vi "Main_09b refactored.vi"() -> ()   [LabVIEW 2020]
uses:
  Cluster_Point.ctl
panel:
  in  "Puzzle Description":string="--- Part Two ---\nA rope snaps! Suddenly, the river is getting a lot closer than you remember. The bridge is still there, but some of the ropes that broke are now whipping toward you as you fall through the air!\n\nThe ropes are moving too quickly to grab; you only have a few seconds to choose how to arch your body to avoid being hit. Fortunately, your simulation can be extended to support longer ropes.\n\nRather than two knots, you now must simulate a rope consisting of ten knots. One knot is still the head of the rope and moves according to the series of motions. Each knot further down the rope follows the knot in front of it using the same rules as before.\n\nUsing the same series of motions as the above example, but with the knots marked H, 1, 2, ..., 9, the motions now occur as follows:\n\n== Initial State ==\n\n......\n......\n......\n......\nH.....  (H covers 1, 2, 3, 4, 5, 6, 7, 8, 9, s)\n\n== R 4 ==\n\n......\n......\n......\n......\n1H....  (1 covers 2, 3, 4, 5, 6, 7, 8, 9, s)\n\n......\n......\n......\n......\n21H...  (2 covers 3, 4, 5, 6, 7, 8, 9, s)\n\n......\n......\n......\n......\n321H..  (3 covers 4, 5, 6, 7, 8, 9, s)\n\n......\n......\n......\n......\n4321H.  (4 covers 5, 6, 7, 8, 9, s)\n\n== U 4 ==\n\n......\n......\n......\n....H.\n4321..  (4 covers 5, 6, 7, 8, 9, s)\n\n......\n......\n....H.\n.4321.\n5.....  (5 covers 6, 7, 8, 9, s)\n\n......\n....H.\n....1.\n.432..\n5.....  (5 covers 6, 7, 8, 9, s)\n\n....H.\n....1.\n..432.\n.5....\n6.....  (6 covers 7, 8, 9, s)\n\n== L 3 ==\n\n...H..\n....1.\n..432.\n.5....\n6.....  (6 covers 7, 8, 9, s)\n\n..H1..\n...2..\n..43..\n.5....\n6.....  (6 covers 7, 8, 9, s)\n\n.H1...\n...2..\n..43..\n.5....\n6.....  (6 covers 7, 8, 9, s)\n\n== D 1 ==\n\n..1...\n.H.2..\n..43..\n.5....\n6.....  (6 covers 7, 8, 9, s)\n\n== R 4 ==\n\n..1...\n..H2..\n..43..\n.5....\n6.....  (6 covers 7, 8, 9, s)\n\n..1...\n...H..  (H covers 2)\n..43..\n.5....\n6.....  (6 covers 7, 8, 9, s)\n\n......\n...1H.  (1 covers 2)\n..43..\n.5....\n6.....  (6 covers 7, 8, 9, s)\n\n......\n...21H\n..43..\n.5....\n6.....  (6 covers 7, 8, 9, s)\n\n== D 1 ==\n\n......\n...21.\n..43.H\n.5....\n6.....  (6 covers 7, 8, 9, s)\n\n== L 5 ==\n\n......\n...21.\n..43H.\n.5....\n6.....  (6 covers 7, 8, 9, s)\n\n......\n...21.\n..4H..  (H covers 3)\n.5....\n6.....  (6 covers 7, 8, 9, s)\n\n......\n...2..\n..H1..  (H covers 4; 1 covers 3)\n.5....\n6.....  (6 covers 7, 8, 9, s)\n\n......\n...2..\n.H13..  (1 covers 4)\n.5....\n6.....  (6 covers 7, 8, 9, s)\n\n......\n......\nH123..  (2 covers 4)\n.5....\n6.....  (6 covers 7, 8, 9, s)\n\n== R 2 ==\n\n......\n......\n.H23..  (H covers 1; 2 covers 4)\n.5....\n6.....  (6 covers 7, 8, 9, s)\n\n......\n......\n.1H3..  (H covers 2, 4)\n.5....\n6.....  (6 covers 7, 8, 9, s)\nNow, you need to keep track of the positions the new tail, 9, visits. In this example, the tail never moves, and so it only visits 1 position. However, be careful: more types of motion are possible than before, so you might want to visually compare your simulated rope to the one above.\n\nHere's a larger example:\n\nR 5\nU 8\nL 8\nD 3\nR 17\nD 10\nL 25\nU 20\nThese motions occur as follows (individual steps are not shown):\n\n== Initial State ==\n\n..........................\n..........................\n..........................\n..........................\n..........................\n..........................\n..........................\n..........................\n..........................\n..........................\n..........................\n..........................\n..........................\n..........................\n..........................\n...........H..............  (H covers 1, 2, 3, 4, 5, 6, 7, 8, 9, s)\n..........................\n..........................\n..........................\n..........................\n..........................\n\n== R 5 ==\n\n..........................\n..........................\n..........................\n..........................\n..........................\n..........................\n..........................\n..........................\n..........................\n..........................\n..........................\n..........................\n..........................\n..........................\n..........................\n...........54321H.........  (5 covers 6, 7, 8, 9, s)\n..........................\n..........................\n..........................\n..........................\n..........................\n\n== U 8 ==\n\n..........................\n..........................\n..........................\n..........................\n..........................\n..........................\n..........................\n................H.........\n................1.........\n................2.........\n................3.........\n...............54.........\n..............6...........\n.............7............\n............8.............\n...........9..............  (9 covers s)\n..........................\n..........................\n..........................\n..........................\n..........................\n\n== L 8 ==\n\n..........................\n..........................\n..........................\n..........................\n..........................\n..........................\n..........................\n........H1234.............\n............5.............\n............6.............\n............7.............\n............8.............\n............9.............\n..........................\n..........................\n...........s..............\n..........................\n..........................\n..........................\n..........................\n..........................\n\n== D 3 ==\n\n..........................\n..........................\n..........................\n..........................\n..........................\n..........................\n..........................\n..........................\n.........2345.............\n........1...6.............\n........H...7.............\n............8.............\n............9.............\n..........................\n..........................\n...........s..............\n..........................\n..........................\n..........................\n..........................\n..........................\n\n== R 17 ==\n\n..........................\n..........................\n..........................\n..........................\n..........................\n..........................\n..........................\n..........................\n..........................\n..........................\n................987654321H\n..........................\n..........................\n..........................\n..........................\n...........s..............\n..........................\n..........................\n..........................\n..........................\n..........................\n\n== D 10 ==\n\n..........................\n..........................\n..........................\n..........................\n..........................\n..........................\n..........................\n..........................\n..........................\n..........................\n..........................\n..........................\n..........................\n..........................\n..........................\n...........s.........98765\n.........................4\n.........................3\n.........................2\n.........................1\n.........................H\n\n== L 25 ==\n\n..........................\n..........................\n..........................\n..........................\n..........................\n..........................\n..........................\n..........................\n..........................\n..........................\n..........................\n..........................\n..........................\n..........................\n..........................\n...........s..............\n..........................\n..........................\n..........................\n..........................\nH123456789................\n\n== U 20 ==\n\nH.........................\n1.........................\n2.........................\n3.........................\n4.........................\n5.........................\n6.........................\n7.........................\n8.........................\n9.........................\n..........................\n..........................\n..........................\n..........................\n..........................\n...........s..............\n..........................\n..........................\n..........................\n..........................\n..........................\n\nNow, the tail (9) visits 36 positions (including s) at least once:\n\n..........................\n..........................\n..........................\n..........................\n..........................\n..........................\n..........................\n..........................\n..........................\n#.........................\n#.............###.........\n#............#...#........\n.#..........#.....#.......\n..#..........#.....#......\n...#........#.......#.....\n....#......s.........#....\n.....#..............#.....\n......#............#......\n.......#..........#.......\n........#........#........\n.........########.........\nSimulate your complete series of motions on a larger rope with ten knots. How many positions does the tail of the rope visit at least once?"
  out "Location array":T1[](array[typedef])
  in  "Example 1":string="R 4\nU 4\nL 3\nD 1\nR 4\nD 1\nL 5\nR 2"
  out "Tail Positon count":i32
  in  "Puzzle":string="R 1\nD 1\nL 1\nD 1\nR 2\nL 1\nU 2\nD 1\nU 2\nL 1\nU 1\nL 2\nD 1\nU 2\nL 1\nR 1\nD 1\nL 2\nD 2\nL 2\nR 1\nL 2\nU 2\nR 2\nL 2\nU 2\nL 1\nD 1\nL 2\nU 1\nR 1\nD 2\nL 2\nU 1\nR 1\nD 1\nU 2\nL 1\nD 2\nU 1\nD 1\nR 2\nD 1\nL 2\nD 1\nL 1\nR 1\nD 2\nL 1\nR 2\nD 2\nU 2\nR 2\nD 2\nR 2\nL 2\nD 2\nL 2\nD 1\nU 2\nR 1\nD 2\nL 2\nR 2\nL 1\nD 1\nU 2\nD 1\nR 2\nU 2\nR 2\nD 1\nL 1\nU 2\nD 1\nU 1\nD 2\nU 1\nR 1\nU 2\nD 1\nL 2\nU 1\nL 2\nD 2\nR 1\nU 2\nL 1\nD 2\nR 1\nU 1\nD 1\nL 2\nU 1\nR 1\nD 2\nU 2\nL 1\nU 2\nD 2\nR 1\nU 2\nR 1\nU 2\nR 1\nD 2\nU 1\nD 2\nL 2\nD 2\nL 2\nD 2\nR 1\nU 1\nD 3\nU 1\nR 2\nU 3\nD 1\nU 2\nD 2\nU 2\nD 1\nU 2\nR 2\nL 2\nU 1\nL 3\nD 1\nR 3\nD 3\nR 2\nL 1\nU 3\nD 1\nU 2\nR 2\nD 1\nR 3\nD 2\nR 3\nD 1\nU 3\nL 3\nR 2\nU 3\nL 3\nU 2\nL 3\nD 1\nR 3\nU 3\nR 2\nD 1\nU 3\nR 3\nD 1\nL 2\nD 2\nL 2\nD 3\nR 2\nU 3\nL 3\nD 2\nU 3\nL 2\nU 3\nD 1\nL 1\nD 3\nR 1\nD 3\nU 1\nL 3\nU 1\nD 2\nU 1\nD 1\nU 2\nD 3\nL 1\nU 1\nR 1\nU 3\nD 3\nR 1\nL 2\nR 3\nL 3\nU 1\nD 2\nR 2\nU 2\nD 3\nU 2\nD 3\nL 1\nR 3\nD 3\nR 2\nU 3\nD 3\nL 2\nR 3\nD 3\nR 2\nL 1\nR 3\nD 2\nR 1\nD 3\nL 1\nU 1\nD 2\nR 1\nD 1\nL 1\nR 2\nL 1\nU 1\nL 2\nD 2\nL 2\nD 1\nL 2\nU 3\nD 1\nR 3\nL 2\nR 1\nL 2\nR 3\nU 2\nL 4\nR 3\nL 1\nR 2\nD 2\nL 4\nU 3\nL 1\nD 1\nL 3\nU 2\nL 3\nU 2\nL 1\nR 2\nL 3\nU 1\nD 2\nR 1\nL 4\nR 4\nL 4\nU 2\nD 2\nR 2\nL 2\nU 2\nR 1\nD 3\nL 4\nR 2\nU 1\nL 4\nR 1\nL 1\nD 4\nR 3\nD 1\nR 2\nL 2\nR 3\nL 1\nU 1\nD 3\nU 2\nR 1\nL 1\nD 3\nR 2\nU 2\nR 3\nU 2\nD 1\nR 4\nU 4\nD 3\nU 3\nR 2\nU 1\nL 1\nU 4\nD 1\nR 4\nD 4\nL 3\nU 4\nR 4\nL 1\nR 1\nU 2\nR 4\nD 2\nR 1\nU 2\nL 1\nD 1\nL 3\nR 3\nL 3\nD 3\nL 4\nD 2\nU 2\nD 3\nR 1\nU 1\nD 3\nU 1\nR 3\nD 2\nL 3\nR 2\nD 1\nL 3\nD 3\nU 3\nD 4\nL 2\nU 3\nD 5\nL 2\nD 2\nR 2\nL 3\nD 5\nU 4\nR 1\nD 5\nR 1\nD 1\nL 2\nR 4\nU 2\nD 3\nR 5\nL 2\nR 2\nD 1\nR 2\nU 5\nL 4\nU 5\nD 1\nL 2\nU 2\nR 2\nD 4\nU 3\nL 2\nD 1\nU 4\nL 4\nD 3\nL 3\nD 3\nR 1\nU 1\nR 1\nU 1\nR 2\nD 3\nR 5\nU 1\nD 2\nL 5\nU 5\nL 4\nD 4\nU 4\nL 1\nR 5\nU 2\nL 3\nU 2\nD 3\nL 5\nD 5\nL 2\nU 2\nD 4\nU 3\nD 3\nL 1\nD 2\nR 2\nD 1\nR 4\nL 3\nD 1\nU 4\nL 1\nR 2\nL 4\nD 5\nR 3\nD 1\nL 5\nD 5\nU 3\nR 2\nD 4\nL 2\nR 2\nD 3\nR 3\nU 2\nR 5\nU 4\nR 3\nL 1\nD 2\nU 1\nL 1\nR 2\nU 4\nD 4\nL 1\nR 1\nU 4\nL 3\nU 5\nR 3\nL 4\nD 3\nU 1\nR 4\nU 1\nL 1\nU 3\nR 4\nL 5\nD 1\nU 4\nR 5\nL 1\nR 4\nD 2\nL 6\nD 5\nU 5\nL 5\nR 6\nD 1\nU 2\nR 1\nU 4\nD 6\nL 6\nD 6\nU 6\nD 4\nU 4\nD 1\nU 3\nL 5\nD 6\nR 1\nL 1\nD 2\nL 4\nD 4\nL 4\nR 4\nU 2\nL 3\nD 4\nR 3\nD 4\nU 5\nR 4\nU 1\nR 6\nL 3\nR 2\nU 1\nL 1\nR 2\nD 3\nR 6\nD 6\nU 1\nD 3\nU 4\nD 5\nL 5\nU 3\nD 6\nL 5\nR 5\nU 1\nR 4\nD 2\nL 2\nR 4\nL 5\nR 4\nL 3\nD 5\nR 6\nL 6\nU 1\nR 5\nU 6\nD 2\nR 2\nD 1\nL 6\nU 4\nL 1\nR 5\nL 1\nR 2\nD 1\nL 4\nU 4\nL 1\nR 3\nU 5\nL 2\nD 6\nU 5\nR 6\nD 6\nU 3\nL 3\nU 3\nL 4\nD 5\nU 2\nD 4\nU 5\nR 6\nU 5\nD 2\nU 6\nD 3\nL 3\nD 6\nL 5\nR 2\nD 6\nR 7\nD 3\nL 7\nD 3\nU 2\nR 7\nU 2\nL 6\nR 7\nD 3\nR 7\nU 5\nR 7\nL 5\nR 7\nL 7\nU 4\nD 4\nU 1\nD 3\nU 1\nD 5\nR 3\nU 1\nD 2\nU 1\nL 4\nU 2\nL 6\nD 7\nU 1\nD 4\nU 6\nL 4\nR 4\nD 4\nR 6\nD 7\nR 1\nD 7\nL 4\nR 4\nL 1\nU 1\nR 6\nL 7\nD 7\nL 5\nU 7\nD 3\nL 6\nD 6\nU 4\nR 1\nL 2\nD 4\nR 3\nL 1\nR 7\nD 1\nL 2\nU 1\nD 2\nR 1\nU 3\nD 4\nL 3\nU 6\nL 4\nR 2\nL 1\nU 6\nD 1\nR 5\nU 2\nD 2\nL 7\nU 2\nR 5\nD 2\nR 4\nD 4\nR 3\nL 2\nR 3\nU 7\nL 5\nR 7\nU 2\nL 7\nD 3\nU 6\nD 4\nU 4\nD 6\nU 3\nL 6\nR 4\nD 2\nR 4\nD 2\nR 3\nL 5\nD 1\nU 7\nD 4\nL 4\nU 2\nD 2\nU 7\nL 5\nR 6\nU 8\nL 7\nD 2\nU 1\nR 6\nD 4\nL 4\nR 7\nD 1\nL 6\nD 7\nR 7\nU 3\nL 6\nU 1\nL 8\nD 6\nU 8\nL 7\nU 5\nD 8\nL 2\nD 3\nL 8\nU 1\nD 5\nL 4\nR 6\nD 8\nL 6\nU 5\nR 3\nU 7\nR 6\nU 3\nL 3\nD 4\nR 4\nL 2\nR 6\nD 3\nR 3\nL 8\nU 2\nD 6\nU 3\nD 8\nU 6\nD 4\nU 8\nR 7\nD 2\nU 6\nD 6\nR 1\nU 3\nD 3\nR 1\nU 3\nR 1\nD 7\nL 8\nR 8\nU 7\nR 3\nL 8\nU 2\nL 8\nD 4\nU 4\nR 1\nD 3\nR 4\nU 3\nL 7\nU 2\nR 7\nD 2\nU 4\nD 3\nL 8\nD 5\nL 3\nU 4\nD 6\nL 5\nD 2\nU 1\nR 6\nL 4\nR 6\nU 5\nR 8\nU 8\nD 7\nL 5\nD 2\nL 8\nU 2\nD 1\nR 1\nL 7\nU 4\nR 2\nU 7\nD 6\nR 6\nL 5\nU 8\nD 7\nR 8\nL 8\nD 6\nU 6\nR 1\nD 5\nL 7\nR 8\nL 4\nD 3\nL 2\nU 5\nR 9\nL 8\nD 8\nL 2\nR 4\nL 7\nR 5\nL 1\nR 8\nD 8\nL 4\nU 2\nD 7\nL 7\nD 6\nR 8\nL 3\nD 7\nU 1\nR 6\nD 6\nU 6\nL 9\nD 1\nR 7\nL 5\nR 5\nU 5\nD 4\nL 8\nU 4\nD 8\nR 4\nD 6\nU 3\nD 7\nL 5\nD 6\nR 9\nU 4\nR 6\nL 3\nU 4\nD 9\nL 7\nR 5\nD 9\nL 6\nU 7\nL 7\nR 4\nD 5\nR 7\nL 5\nR 3\nU 8\nL 6\nU 5\nL 9\nR 8\nU 4\nD 2\nL 4\nD 7\nR 7\nD 4\nL 4\nU 2\nL 3\nR 1\nD 3\nU 6\nR 1\nU 8\nR 2\nL 4\nD 3\nL 5\nU 4\nR 7\nL 2\nR 7\nL 9\nD 9\nU 5\nL 4\nU 1\nD 1\nU 6\nD 1\nL 6\nD 7\nU 5\nD 9\nR 9\nD 5\nU 9\nL 3\nR 5\nD 10\nR 1\nU 7\nD 6\nL 3\nU 5\nR 1\nD 5\nR 8\nU 3\nL 1\nD 2\nR 1\nL 6\nR 8\nD 9\nU 9\nD 4\nR 1\nU 8\nL 5\nU 4\nD 7\nL 1\nR 4\nL 6\nD 4\nR 5\nD 1\nR 10\nD 5\nR 7\nU 6\nR 5\nU 2\nL 8\nR 1\nU 3\nL 5\nU 4\nL 3\nD 3\nU 6\nD 10\nL 3\nD 7\nL 5\nD 4\nU 6\nR 9\nU 5\nD 5\nR 2\nL 7\nU 8\nD 5\nR 9\nL 6\nR 8\nU 9\nL 4\nR 10\nD 10\nL 9\nR 8\nL 4\nR 5\nL 9\nD 1\nL 3\nR 9\nU 2\nL 5\nR 2\nU 1\nR 4\nD 10\nU 3\nD 8\nL 9\nD 8\nL 5\nD 4\nU 2\nL 8\nR 5\nU 4\nD 1\nL 4\nU 7\nD 9\nR 3\nD 7\nR 9\nL 6\nR 6\nU 8\nL 10\nU 5\nD 4\nR 5\nL 6\nD 7\nL 10\nR 1\nL 9\nU 6\nD 9\nR 7\nL 7\nD 6\nU 6\nR 1\nD 7\nL 1\nR 9\nD 9\nR 3\nL 5\nD 4\nR 3\nL 5\nD 11\nU 1\nR 6\nD 8\nR 4\nD 3\nR 9\nU 3\nD 8\nU 7\nR 2\nU 10\nR 4\nL 4\nD 10\nR 8\nU 11\nR 7\nD 7\nR 9\nD 11\nU 6\nR 7\nD 10\nL 4\nD 5\nL 7\nD 3\nL 4\nD 4\nU 4\nR 3\nL 9\nD 4\nL 8\nU 5\nR 7\nL 2\nD 4\nR 11\nU 10\nD 3\nR 8\nD 3\nR 10\nL 8\nU 6\nR 4\nD 10\nR 7\nD 3\nR 2\nU 1\nD 5\nL 8\nU 2\nR 1\nU 8\nR 11\nL 3\nU 10\nL 5\nD 3\nL 6\nU 10\nL 11\nD 4\nL 5\nD 1\nL 4\nD 1\nL 3\nR 7\nU 7\nR 4\nL 1\nU 10\nD 11\nL 1\nR 1\nU 9\nD 6\nL 9\nD 1\nL 4\nD 11\nL 5\nU 2\nL 5\nD 8\nU 10\nD 5\nU 10\nL 8\nR 11\nD 10\nU 11\nR 4\nU 6\nD 11\nR 1\nL 4\nU 12\nL 8\nU 12\nD 4\nL 7\nU 7\nL 8\nD 3\nU 1\nL 12\nD 5\nU 3\nD 6\nR 7\nU 1\nD 12\nR 6\nU 3\nD 3\nR 12\nU 5\nR 3\nU 8\nL 6\nR 6\nU 3\nL 4\nD 8\nL 5\nD 12\nU 1\nL 9\nR 4\nL 1\nD 6\nU 9\nL 5\nR 3\nL 9\nD 8\nR 6\nD 3\nU 6\nL 1\nD 7\nU 5\nD 1\nL 11\nR 7\nD 11\nL 3\nU 6\nR 9\nD 12\nR 11\nL 5\nR 8\nL 2\nU 10\nR 6\nU 10\nL 9\nU 1\nL 1\nR 8\nL 7\nR 3\nU 4\nL 3\nR 8\nL 9\nR 11\nL 9\nD 11\nU 1\nL 12\nR 6\nL 3\nR 3\nD 12\nU 9\nL 9\nD 8\nR 4\nL 7\nR 1\nU 2\nR 4\nU 4\nR 11\nU 7\nD 11\nU 3\nD 6\nU 7\nL 2\nD 4\nU 9\nR 3\nL 8\nR 9\nL 4\nR 5\nL 7\nD 3\nR 8\nL 6\nU 10\nR 3\nL 6\nD 8\nU 3\nD 9\nL 1\nU 13\nR 12\nL 13\nR 2\nU 8\nR 1\nD 11\nR 5\nL 4\nU 5\nL 3\nD 13\nU 2\nD 1\nU 2\nL 9\nD 3\nR 6\nU 13\nL 3\nU 5\nR 2\nD 2\nL 5\nU 4\nR 6\nD 1\nU 9\nL 7\nR 11\nU 10\nD 12\nR 10\nU 7\nR 5\nL 2\nR 13\nL 13\nD 3\nR 7\nU 1\nL 1\nD 2\nL 9\nU 12\nD 7\nU 13\nL 12\nU 13\nD 7\nU 7\nD 8\nL 2\nU 6\nD 2\nU 6\nL 8\nU 4\nD 11\nU 11\nL 11\nR 10\nL 10\nR 6\nD 13\nU 2\nL 7\nU 8\nD 1\nR 6\nL 7\nR 9\nL 8\nR 9\nL 6\nR 7\nD 12\nR 11\nL 8\nR 1\nD 5\nR 5\nL 10\nU 6\nL 8\nD 9\nL 5\nU 4\nD 12\nU 8\nL 13\nU 6\nD 10\nR 5\nL 13\nD 7\nL 13\nR 5\nL 10\nD 13\nL 9\nR 3\nD 8\nU 9\nD 10\nU 10\nD 7\nL 5\nR 5\nD 9\nL 7\nR 10\nD 13\nR 1\nU 2\nR 6\nU 14\nR 10\nD 6\nU 13\nD 14\nU 5\nD 1\nU 8\nR 4\nU 9\nR 13\nL 4\nD 2\nR 8\nU 2\nD 12\nU 3\nR 6\nU 6\nD 11\nR 7\nL 12\nR 9\nU 7\nD 1\nR 14\nL 11\nU 4\nD 13\nU 5\nL 7\nR 14\nL 1\nU 6\nD 3\nL 1\nU 13\nD 8\nU 14\nD 5\nU 14\nL 1\nR 1\nD 5\nU 7\nL 8\nR 6\nU 1\nD 2\nR 14\nU 13\nL 10\nU 8\nD 13\nU 6\nR 2\nD 4\nR 6\nU 7\nD 10\nL 6\nU 5\nL 3\nD 9\nU 13\nD 8\nU 3\nR 3\nL 12\nD 5\nR 8\nU 7\nR 11\nU 6\nD 7\nR 13\nU 1\nD 9\nU 10\nD 3\nL 5\nR 12\nL 4\nD 13\nR 7\nD 12\nR 11\nD 9\nR 5\nU 13\nR 3\nD 4\nU 10\nR 3\nU 6\nL 4\nR 1\nU 4\nL 9\nD 11\nU 5\nD 3\nU 13\nD 1\nL 1\nD 13\nL 2\nR 9\nL 4\nR 2\nU 9\nD 9\nU 12\nL 14\nR 2\nL 9\nR 5\nU 2\nD 3\nR 13\nU 5\nD 1\nU 15\nR 6\nD 14\nR 8\nL 9\nD 14\nL 6\nR 8\nU 14\nR 11\nL 3\nD 15\nU 5\nR 1\nL 7\nR 12\nD 1\nR 4\nD 13\nU 9\nD 2\nL 3\nU 10\nR 10\nD 2\nR 6\nU 13\nD 7\nR 5\nU 5\nL 12\nU 6\nR 1\nL 7\nU 9\nD 15\nL 8\nU 9\nL 5\nR 3\nL 9\nU 6\nL 11\nD 8\nL 11\nD 13\nU 3\nR 6\nD 2\nL 10\nR 15\nU 2\nD 8\nR 6\nD 6\nL 8\nD 7\nU 2\nD 14\nU 4\nR 6\nD 15\nL 12\nR 4\nD 3\nU 7\nD 10\nL 8\nU 7\nR 10\nU 11\nD 2\nR 10\nD 10\nU 13\nR 8\nL 2\nU 12\nR 9\nU 12\nR 5\nU 10\nL 6\nR 3\nD 10\nL 10\nU 6\nL 4\nR 3\nD 9\nR 15\nD 14\nL 11\nR 5\nU 2\nR 14\nL 15\nR 3\nD 3\nL 4\nU 10\nD 14\nL 9\nD 5\nL 16\nU 12\nL 4\nD 15\nL 10\nR 14\nD 4\nR 12\nL 7\nU 5\nR 3\nL 6\nU 16\nL 5\nU 8\nD 8\nL 6\nD 3\nU 14\nR 1\nL 13\nU 4\nD 11\nR 5\nL 11\nD 7\nR 1\nL 14\nU 10\nL 5\nD 15\nU 14\nL 4\nD 7\nU 3\nR 1\nU 2\nR 3\nD 16\nU 7\nR 7\nD 13\nR 7\nD 5\nU 7\nR 16\nU 4\nL 3\nR 9\nU 1\nD 2\nR 5\nD 3\nU 8\nR 5\nL 13\nU 13\nL 2\nR 9\nL 14\nD 10\nR 1\nU 1\nR 14\nU 14\nR 2\nL 1\nR 12\nL 1\nD 6\nR 2\nD 7\nR 11\nL 5\nD 8\nR 15\nD 12\nR 12\nL 8\nD 10\nR 2\nD 12\nU 15\nL 9\nD 4\nU 3\nL 8\nD 3\nU 9\nD 16\nL 2\nU 14\nR 15\nD 14\nU 12\nD 6\nU 14\nR 11\nD 12\nR 2\nU 13\nL 2\nR 1\nD 6\nU 13\nD 15\nU 1\nR 14\nL 16\nD 8\nR 13\nL 14\nR 3\nD 8\nL 6\nR 16\nD 6\nL 13\nR 2\nL 11\nD 2\nU 1\nR 15\nL 9\nU 1\nR 12\nL 9\nD 7\nL 8\nU 2\nL 14\nR 7\nU 8\nD 15\nR 8\nD 13\nL 15\nR 11\nD 17\nU 2\nR 14\nL 9\nU 11\nD 6\nU 4\nD 8\nU 16\nD 5\nL 3\nD 11\nL 7\nU 11\nL 4\nD 5\nL 5\nD 2\nU 8\nR 17\nD 17\nU 12\nR 4\nL 13\nR 15\nL 10\nU 2\nL 10\nR 6\nD 1\nU 6\nL 3\nD 8\nR 4\nD 1\nL 4\nD 13\nR 1\nU 3\nL 1\nU 9\nD 13\nU 2\nD 13\nR 6\nD 8\nR 6\nD 13\nR 4\nD 10\nL 10\nU 8\nD 1\nR 6\nU 14\nR 3\nL 10\nU 15\nL 11\nU 13\nL 4\nU 5\nL 16\nR 16\nU 11\nR 14\nD 7\nU 5\nR 9\nL 5\nU 12\nR 16\nU 10\nD 5\nR 17\nL 3\nD 5\nU 13\nR 3\nU 3\nL 14\nU 1\nL 8\nR 2\nD 3\nU 9\nD 7\nL 1\nD 5\nR 16\nD 12\nR 1\nU 2\nL 16\nU 3\nR 18\nD 11\nR 3\nL 17\nR 7\nL 6\nD 13\nL 5\nR 12\nD 3\nU 1\nL 1\nU 5\nL 8\nR 11\nL 13\nD 14\nR 17\nD 17\nL 2\nU 7\nD 18\nR 3\nD 2\nU 6\nD 9\nR 3\nU 3\nR 5\nD 16\nR 9\nD 13\nU 8\nD 17\nR 4\nL 6\nR 7\nD 2\nR 15\nU 10\nR 15\nD 6\nL 8\nR 17\nD 5\nL 9\nU 18\nD 10\nU 3\nL 6\nU 10\nD 10\nU 16\nR 6\nD 18\nU 10\nD 8\nU 14\nR 3\nU 14\nL 16\nR 3\nD 5\nL 2\nR 4\nD 9\nL 13\nR 17\nL 8\nD 2\nR 16\nD 18\nL 11\nD 15\nU 5\nD 7\nU 14\nD 13\nU 7\nL 13\nD 13\nR 1\nD 15\nR 11\nL 1\nU 6\nD 14\nL 6\nU 8\nD 15\nR 8\nL 12\nD 17\nR 8\nL 17\nD 16\nR 9\nD 19\nU 4\nR 9\nU 10\nL 3\nU 3\nD 5\nR 2\nU 6\nL 16\nD 8\nR 4\nL 16\nR 15\nU 6\nL 8\nD 6\nL 6\nR 1\nL 8\nD 13\nL 1\nU 7\nR 16\nL 16\nU 1\nL 18\nD 16\nL 8\nU 2\nD 1\nR 2\nD 10\nU 8\nD 2\nR 18\nU 14\nD 15\nR 15\nU 3\nD 1\nU 17\nL 17\nD 15\nL 14\nR 6\nL 18\nU 19\nL 6\nU 17\nL 1\nD 2\nU 17\nR 11\nL 3\nR 3\nL 12\nU 1\nL 9\nU 13\nD 15\nU 12\nR 1\nL 5\nD 17\nL 14\nD 13\nL 2\nD 10\nU 5\nR 13\nL 19\nD 1\nR 12\nU 17\nR 15\nD 19\nU 12\nD 16\nR 2\nU 3\nR 15\nL 13\nU 11\nD 19\nR 10\nD 19\nL 2\nU 12\nR 5\nL 13\nU 13\nR 1\nD 11\nR 17\nD 7\nU 4\nD 14\nL 13\nR 8\nL 8\nD 8"
  in  "Example 2":string="R 5\nU 8\nL 8\nD 3\nR 17\nD 10\nL 25\nU 20"
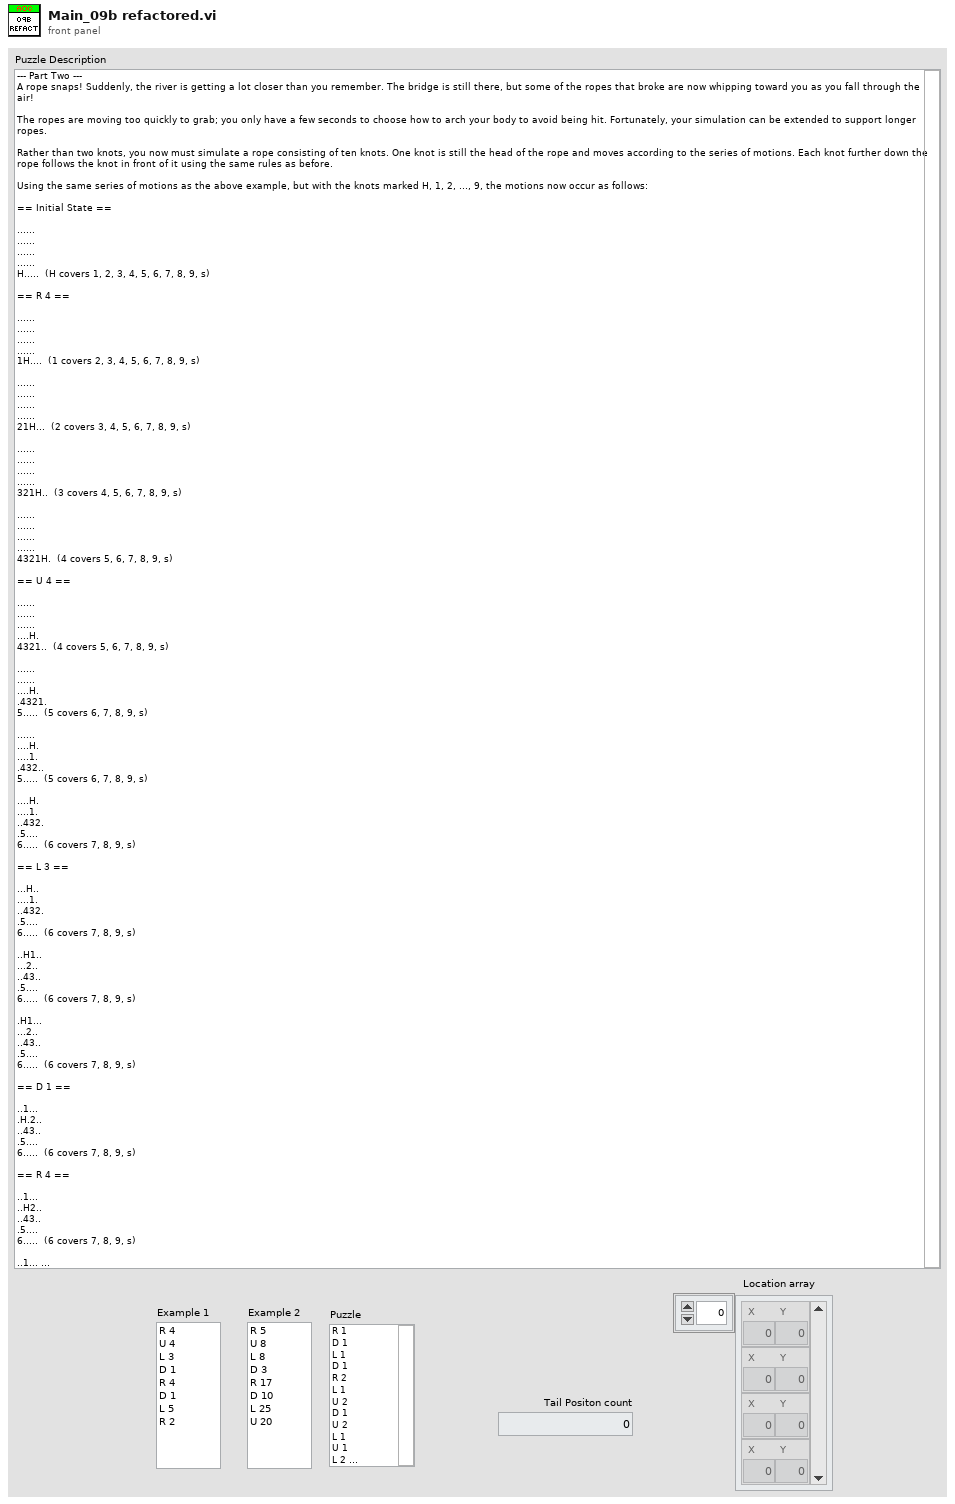
[diagram p1: front panel]
types:
  T1 = typedef "Cluster_Point.ctl" = cluster{"X":i32, "Y":i32}
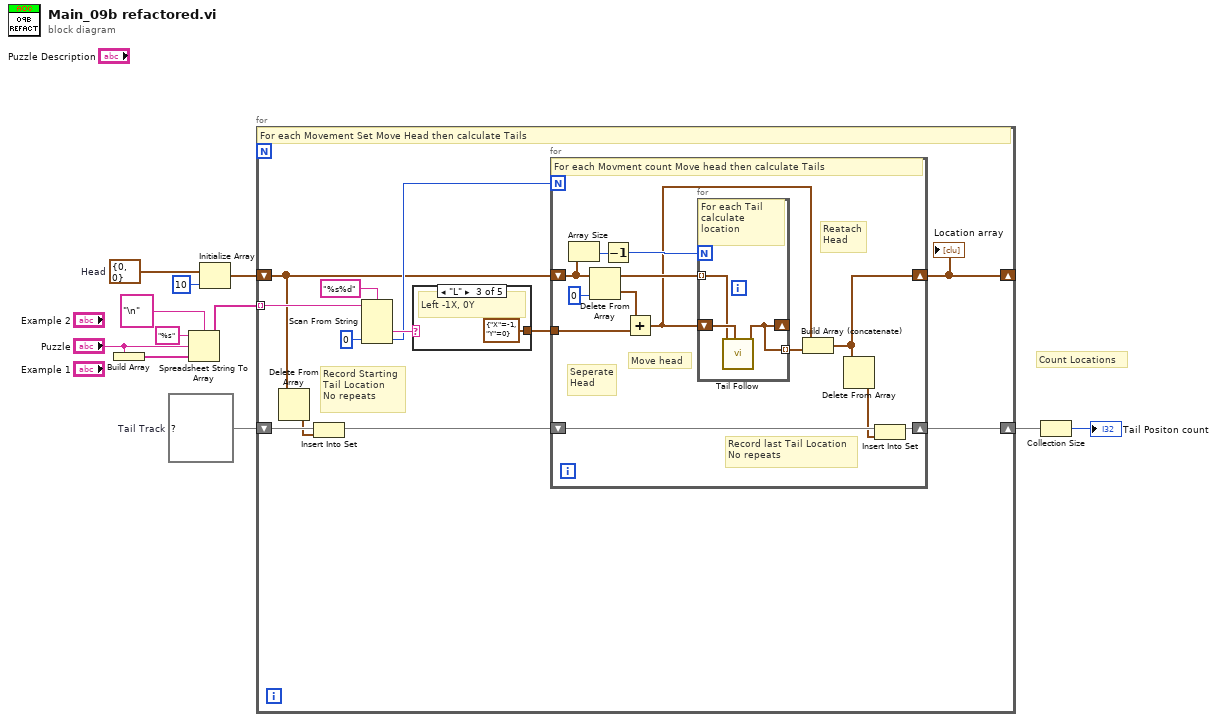
[diagram p0: block diagram]
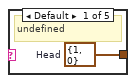
[diagram p2: hidden frame]
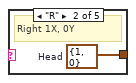
[diagram p3: hidden frame]
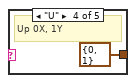
[diagram p4: hidden frame]
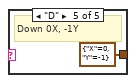
[diagram p5: hidden frame]
diagram:
  w3 = T1 {"X"=0, "Y"=0}  # Head
  w7 = set{T1} {}  # Tail Track
  # "Count Locations"
  n1 = Build Array("Puzzle") -> (w11:string[])
  n2 = Spreadsheet String To Array(delimiter (Tab)="\n", format string="%s", spreadsheet string="Puzzle", array type (2D Dbl)=w11) -> (array=w8:string[])
  n3 = Initialize Array(w3, 10 ("dimension size")) -> (w2:T1[])
  n4 = for {
    tunnel: w8 -> [w22] mode=indexing
    shift-right: [w18] -> w6
    shift-left: w7 -> [w16]
    shift-right: [w12] -> _
    shift-left: w2 -> [w14]
    # "Record Starting\nTail Location\nNo repeats"
    # "For each Movement Set Move Head then calculate Tails"
    n5 = Delete From Array(array=w14) -> (deleted portion=w13:T1)  [unwired: 2 in, 1 out]
    n6 = Insert Into Set(10:w13, 11:w16) -> (3:w15:set{T1})  [unwired: 1 out]
    n7 = Scan From String(format string="%s%d", input string=w22, default 2=0 ("default value 2")) -> (output 1=w21:string, output 2=w19:i32)  [unwired: 3 in, 3 out]
    n8 = case shown="\"L\"" w21 {
      tunnel: [w40 w41 T1 {"X"=-1, "Y"=0} ("Head") T1 {"X"=0, "Y"=1} ("Head") T1 {"X"=0, "Y"=-1} ("Head")] -> w17
      frame Default {
        w40 = T1 {"X"=1, "Y"=0}  # Head
        # "undefined"
      }
      frame "R" {
        w41 = T1 {"X"=1, "Y"=0}  # Head
        # "Right 1X, 0Y"
      }
      frame "L" {
        # "Left -1X, 0Y"
      }
      frame "U" {
        # "Up 0X, 1Y"
      }
      frame "D" {
        # "Down 0X, -1Y"
      }
    }
    n9 = for {
      N: w19 -> [_]
      shift-right: [w35] -> w18
      shift-left: w15 -> [w36]
      tunnel: w17 -> [w30]
      shift-right: [w26] -> w12
      shift-left: w14 -> [w32]
      # "Seperate\nHead"
      # "Reatach\nHead"
      # "Record last Tail Location\nNo repeats"
      # "Move head"
      # "For each Movment count Move head then calculate Tails"
      n10 = Array Size(array=w32) -> (size(s)=w34:i32)
      n11 = Delete From Array(array=w32, index=0) -> (deleted portion=w29:T1, array with subset deleted=w31:T1[])  [unwired: 1 in]
      n12 = Decrement(x=w34) -> (x-1=w33:i32)
      n13 = Add(x=w29, y=w30) -> (x+y=w25:T1)
      n14 = for {
        N: w33 -> [_]
        shift-right: [w37] -> _
        shift-left: w25 -> [w39]
        tunnel: w31 -> [w38] mode=indexing
        tunnel: [w37] -> w28 mode=indexing
        # "For each Tail calculate location"
        n15 = call "Tail Follow.vi"("Head"=w39, "Tail"=w38) -> ("Tail Out"=w37:T1)  [unwired: 9 in]
      }
      n16 = Build Array (concatenate)(w25, w28) -> (w26:T1[])
      n17 = Delete From Array(array=w26) -> (deleted portion=w27:T1)  [unwired: 2 in, 1 out]
      n18 = Insert Into Set(10:w27, 11:w36) -> (3:w35:set{T1})  [unwired: 1 out]
    }
    "Location array" <- w12
  }
  n19 = Collection Size(1:w6) -> (0:→"Tail Positon count":i32)
